vi "GetMarkerName.vi"(8 "error in (no error)":errorcluster, 11 "Keysight44xx in":refnum<class "Keysight44xx.lvclass">) -> (0 "error out":errorcluster, 2 "MarkerName(s)":string[](array[string]), 3 "Keysight44xx out":refnum<class "Keysight44xx.lvclass">)   [LabVIEW 2018, in "SpecAnPlugins.lvlib" / "Keysight44xx.lvclass"]
uses:
  Keysight44xx.lvclass
  C:/Users/ico/Documents/Projects/NistPluggableModules/SpecAn/SpecAnPlugins/SpecAnBaseClass/SpecAnBase.lvclass
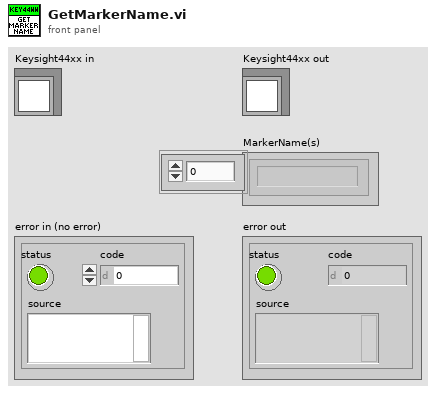
[diagram p1: front panel]
types:
  T1 = typedef "SpecAnPlugins.lvlib/SpecAnBase.lvclass/Acquisition.ctl" = cluster{"Handle":string, "Connected":bool, "Enabled":bool, "SweepModeContinuous":bool, "NumberOfSweeps":i32, "DetectorTypeAuto":bool, "DetectorType":i32, "VerticalScale":i32, "MaximumTime(seconds)":dbl}
  T2 = typedef "SpecAnPlugins.lvlib/SpecAnBase.lvclass/Trace.ctl" = cluster{"TraceName":string, "TraceSize":i32, "TraceType":i32}[]
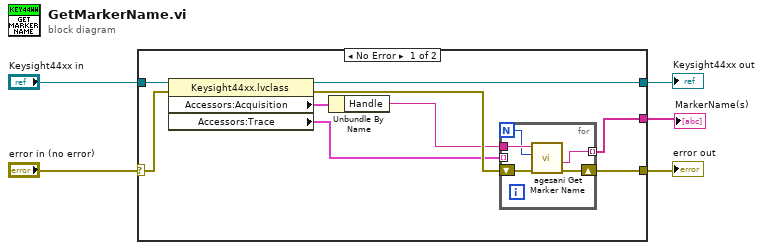
[diagram p0: block diagram]
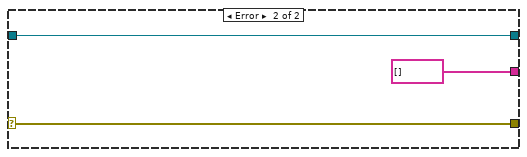
[diagram p2: hidden frame]
diagram:
  n1 = case shown="No Error" "error in (no error)" {
    selector: "error in (no error)" -> [w13 w21]
    tunnel: [w10 w21] -> w4
    tunnel: "Keysight44xx in" -> [w14 w22]
    tunnel: [w12 w22] -> w2
    tunnel: [w7 string[] []] -> w1
    frame No Error {
      n2 = property class="Keysight44xx.lvclass"(reference=w14, error in=w13) -> (reference out=w12:refnum<class "Keysight44xx.lvclass">, error out=w11:errorcluster, "Accessors:Acquisition"=w9:T1, "Accessors:Trace"=w6:T2)
      n3 = Unbundle By Name(w9) -> ("Handle"=w8:string)
      n4 = for {
        N -> [w15]
        tunnel: w8 -> [w17]
        shift-right: [w18] -> w10
        shift-left: w11 -> [w19]
        tunnel: [w16] -> w7 mode=indexing
        tunnel: w6 -> [_] mode=indexing
        n5 = call <instrlib>:"agesani Get Marker Name.vi"("error in (no error)"=w19, "index"=w15, "instrument handle"=w17) -> ("error out"=w18:errorcluster, "name"=w16:string)  [unwired: 6 in, 1 out]
      }
    }
    frame Error {
    }
  }
  "error out" <- w4
  "Keysight44xx out" <- w2
  "MarkerName(s)" <- w1
